vi "Voltage and Current Ring Chooser.vi"(8 "error in (no error)":errorcluster, 11 "Tektronix DMM4020 in":refnum<class "Tektronix DMM4020.lvclass">) -> (0 "error out":errorcluster, 3 "Tektronix DMM4020 out":refnum<class "Tektronix DMM4020.lvclass">)   [LabVIEW 2014, in "Tektronix DMM4020.lvclass"]
uses:
  Tektronix DMM4020.lvclass
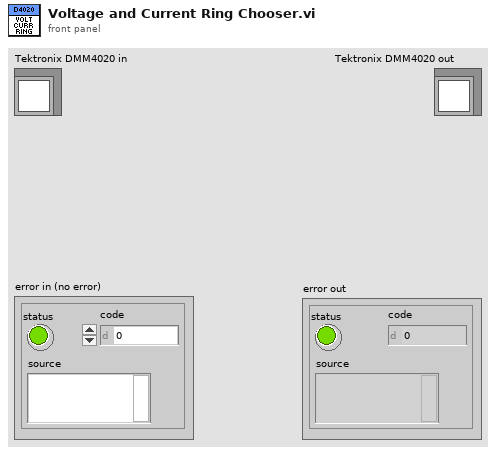
[diagram p1: front panel]
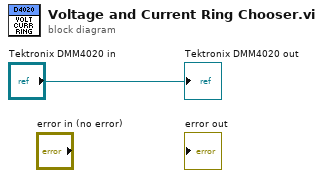
[diagram p0: block diagram]
diagram:
  "Tektronix DMM4020 out" <- "Tektronix DMM4020 in"
